vi "Func_SetConstValue.vi"(8 "error in (no error)":errorcluster, 10 "Number of Items":u32, 11 "VI's Path":path) -> (0 "error out":errorcluster)   [LabVIEW 2010, in "TemplateGenerator.lvlib"]
uses:
  TemplateGenerator.lvlib
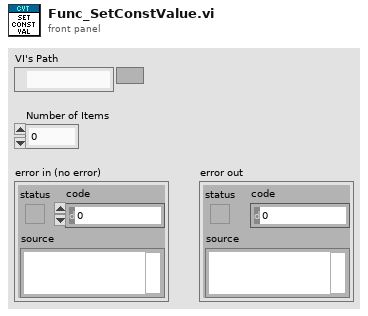
[diagram p1: front panel]
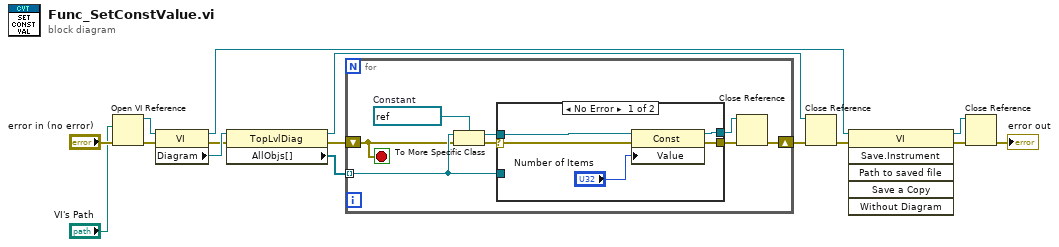
[diagram p0: block diagram]
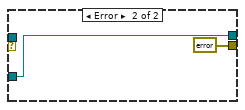
[diagram p2: hidden frame]
diagram:
  n1 = Open VI Reference(vi path="VI's Path", error in (no error)="error in (no error)") -> (vi reference=w7:refnum<vi>, error out=w6:errorcluster)  [unwired: 4 in]
  n2 = property class="VI"(reference=w7, error in=w6) -> (reference out=w2:refnum<vi>, error out=w8:errorcluster, "Diagram"=w9:refnum<vi>)
  n3 = property class="TopLvlDiag"(reference=w9, error in=w8) -> (reference out=w13:refnum<vi>, error out=w10:errorcluster, "AllObjs[]"=w11:refnum<vi>[])
  n4 = for {
    tunnel: w11 -> [w20] mode=indexing
    shift-right: [w17] -> w12
    shift-left: w10 -> [w16]
    stop <- w16 stop-if-true
    w23 = refnum<vi> refnum  # Constant
    n5 = To More Specific Class(target class=w23, reference=w20, error in=w16) -> (specific class reference=w21:refnum<vi>, error out=w22:errorcluster)
    n6 = case shown="No Error" w22 {
      selector: w22 -> [w27 _]
      tunnel: w21 -> [w28 _]
      tunnel: w20 -> [_ w30]
      tunnel: [w26 w30] -> w19
      tunnel: [w25 errorcluster {"status"=FALSE, "code"=0, "source"=""} ("error out")] -> w18
      frame No Error {
        n7 = property class="Const"(reference=w28, error in=w27, "Value"="Number of Items") -> (reference out=w26:refnum<vi>, error out=w25:errorcluster)
      }
      frame Error {
      }
    }
    n8 = Close Reference(reference=w19, error in (no error)=w18) -> (error out=w17:errorcluster)
  }
  n9 = Close Reference(reference=w13, error in (no error)=w12) -> (error out=w5:errorcluster)
  n10 = invoke class="VI" method="Save.Instrument"(reference=w2, error in=w5) -> (reference out=w4:refnum<vi>, error out=w3:errorcluster)  [unwired: 4 in, 4 out]
  n11 = Close Reference(reference=w4, error in (no error)=w3) -> (error out=→"error out":errorcluster)
